vi "Cache-GEvt Refs.vi"(8 "error in (no error)":errorcluster) -> (0 "error out":errorcluster, 3 "CSM Global Log Ref":T1)   [LabVIEW 2017, in "Communicable State Machine.lvlib"]
uses:
  Communicable State Machine.lvlib
  GEvt-Refs.ctl
  Typedef/_CSM_GlobalLog_MSG.ctl
  Typedef/_CSM_Response Source Message.ctl
  Typedef/_CSM_GlobalLog_MSG_TYPE.ctl
  ChangeFlag/ChangeFlag-Read.vi
  ChangeFlag/ChangeFlagDB.vi
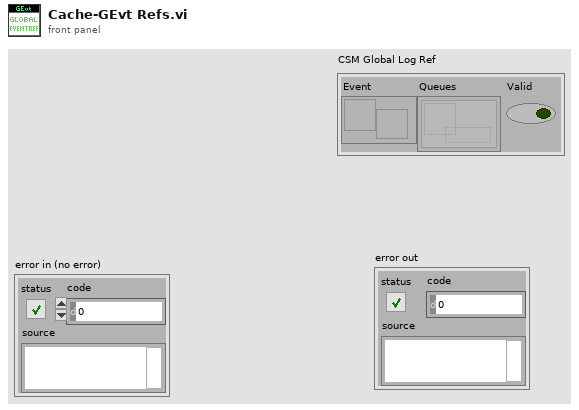
[diagram p1: front panel]
types:
  T1 = typedef "Communicable State Machine.lvlib/GEvt-Refs.ctl" = cluster{"Event":refnum<user-event>, "Queues":refnum<queue>[], "Valid":bool}
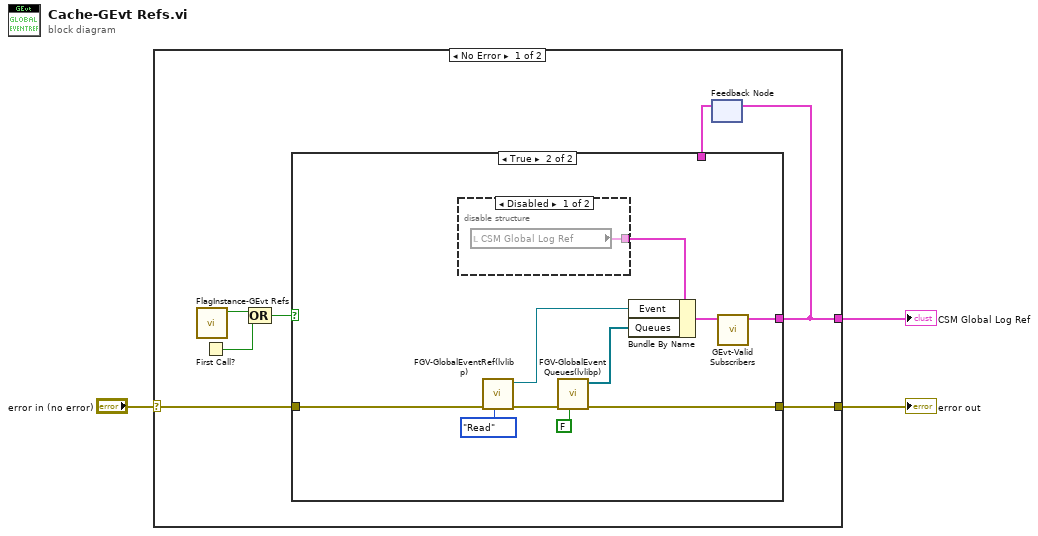
[diagram p0: block diagram]
diagram:
  n1 = case shown="No Error" "error in (no error)" {
    selector: "error in (no error)" -> [w10 w24]
    tunnel: [w6 _] -> w3
    tunnel: [w9 w24] -> w1
    frame No Error {
      n2 = call "FlagInstance-GEvt Refs.vi"() -> ("Changed"=w4:bool)  [unwired: 10 in, 1 out]
      n3 = First Call?() -> (First Call?: T/F=w8:bool)
      n4 = Compound Arithmetic op=OR(w4, w8) -> (w7:bool)
      n5 = feedback #1() -> (w5:T1)  [unwired: 1 in]
      n6 = case shown="True" w7 {
        tunnel: [w12 w18] -> w6
        tunnel: w10 -> [w11 w20]
        tunnel: [w11 w16] -> w9
        tunnel: w5 -> [w12 _]
        frame False {
        }
        frame True {
          n7 = disable-structure shown="Disabled" {
            disable-tunnel: [w23 _] -> w22
            frame Disabled {
              n8 = local read "CSM Global Log Ref"() -> (w23:T1)
            }
            frame Enabled {
            }
          }
          n9 = call "FGV-GlobalEventRef(lvlibp).vi"("Operation"=enum16{"Create", "Read", "Destroy"}."Read", "error in (no error)"=w20) -> ("error out"=w17:errorcluster, "Event"=w21:refnum<user-event>)  [unwired: 8 in]
          n10 = call "FGV-GlobalEventQueues(lvlibp).vi"("Create? (F)"=FALSE, "error in (no error)"=w17) -> ("error out"=w16:errorcluster, "Queue"=w15:refnum<queue>[])  [unwired: 7 in, 1 out]
          n11 = Bundle By Name(cluster=w22, "Event"=w21, "Queues"=w15) -> (w19:T1)
          n12 = call "GEvt-Valid Subscribers.vi"("CSM Global Log Event In"=w19) -> ("CSM Global Log Event Out"=w18:T1)  [unwired: 9 in, 1 out]
        }
      }
      n13 = feedback-in #1(w6) -> ()
    }
    frame Error {
    }
  }
  "CSM Global Log Ref" <- w3
  "error out" <- w1
